vi "niFpga wdp fft output buffer dummy.vi"(4 "enable":bool, 6 "memory switch":bool, 8 "read index":fxp<+,9,9>, 9 "write index":fxp<+,9,9>, 10 "data in 1":T1, 11 "data in 0":T1) -> (2 "data out im":fxp<+/-,32,16>[](array[numeric]), 3 "data out re":fxp<+/-,32,16>[](array[numeric]))   [LabVIEW 2017]
types:
  T1 = cluster{"data re":fxp<+/-,19,1>, "data im":fxp<+/-,19,1>}
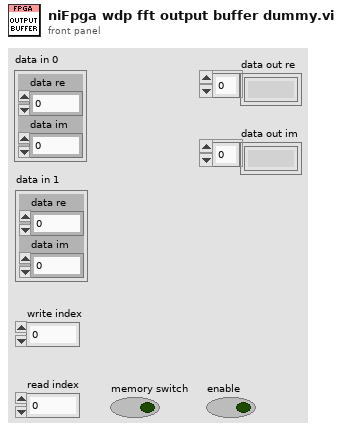
[diagram p1: front panel]
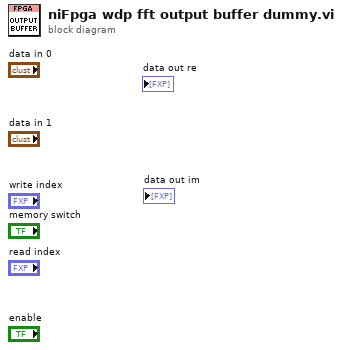
[diagram p0: block diagram]
diagram:
